vi "SubVI_ShowIncorrectImg_002.vi"(1 "output cluster":T1, 2 "selected path":path[](array[path]), 3 "Correct?":bool[](array[boolean])) -> (0 "This VI":refnum<vi>)   [LabVIEW 2018]
uses:
  <vilib>/picture/picture.llb/Draw 1-Bit Pixmap.vi
panel:
  in  "Close This Window":bool
  out "File name":string[](array[string])
  out "Result given":string[](array[string])
  out "Uncorrectly classified pics":picture[](array[picture])
  in  "Just an empty square. Look away!":picture
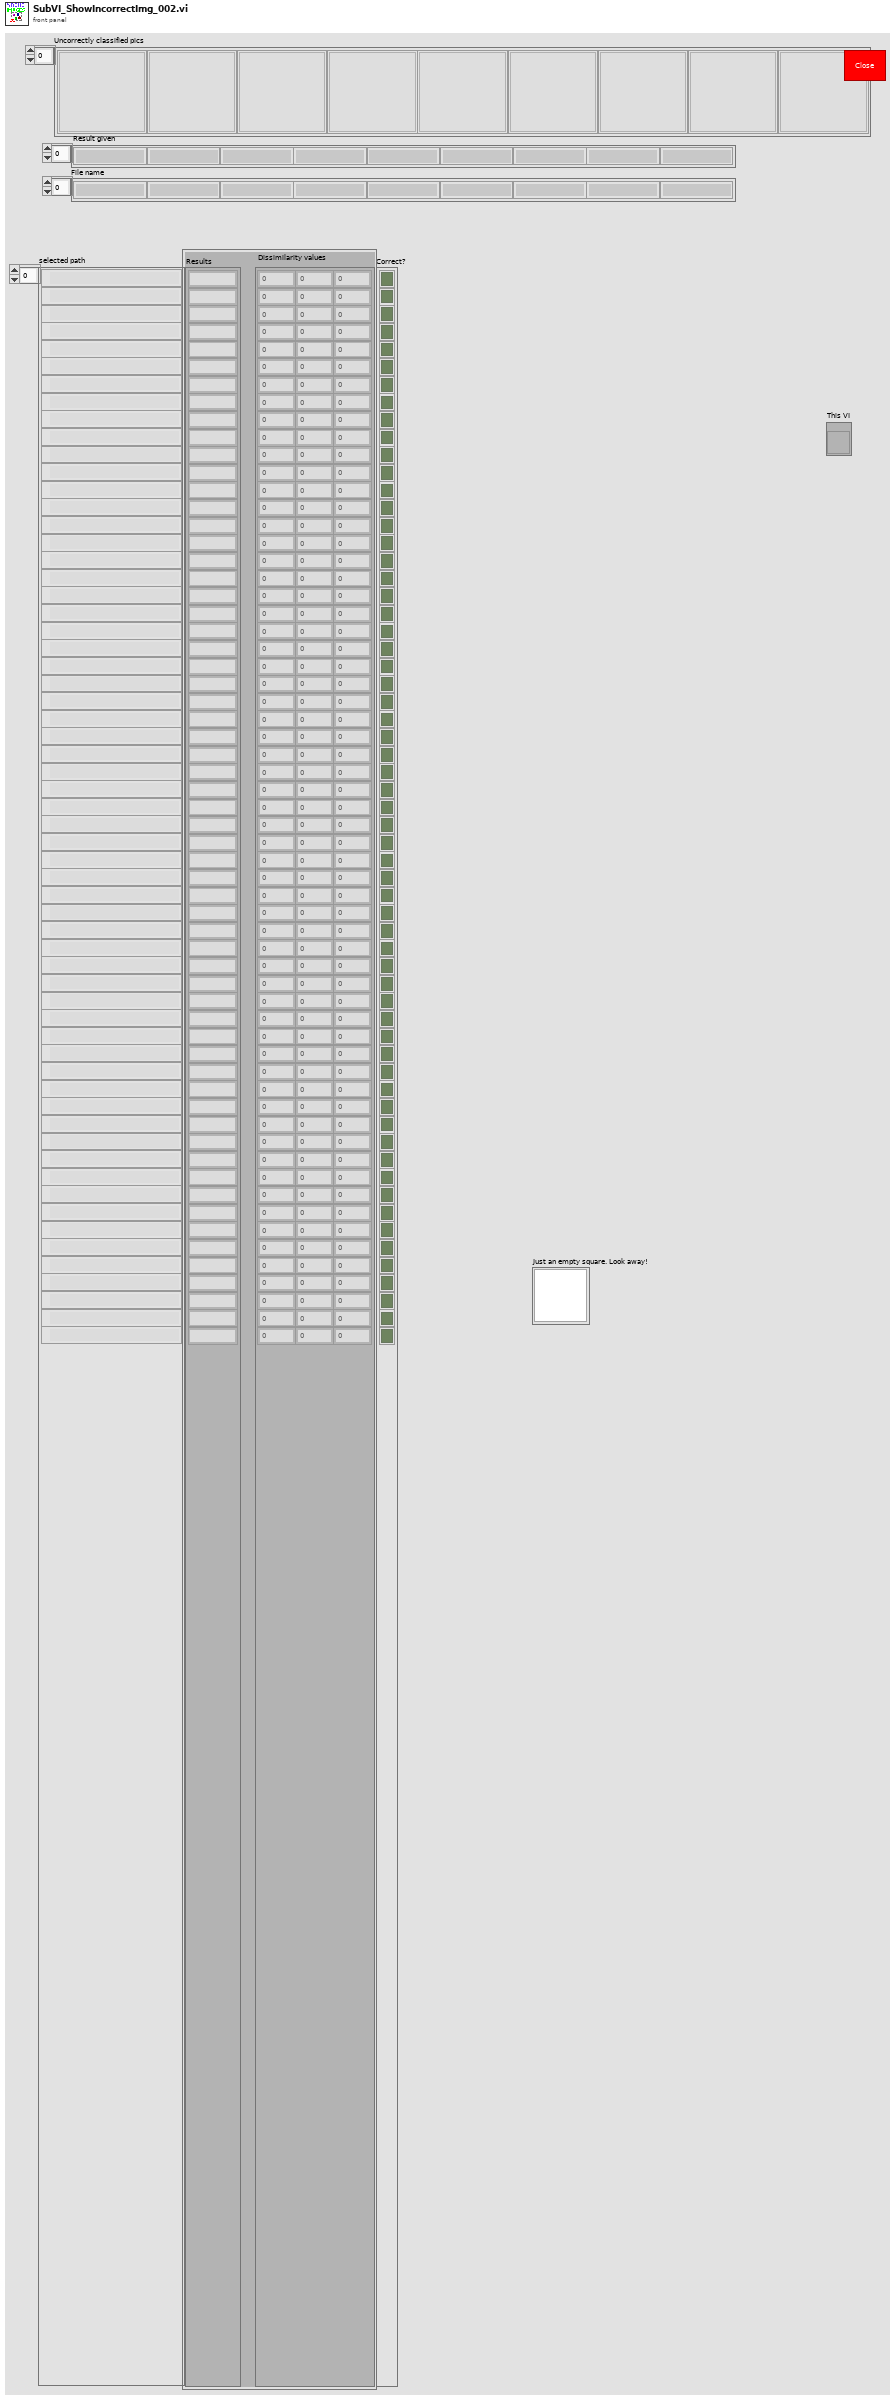
[diagram p1: front panel]
types:
  T1 = cluster{"Results":string[], "Dissimilarity values":dbl[][]}
  T2 = typedef "imagedata.ctl" = cluster{"image type":i32, "image depth":i32, "image":u8[], "mask":u8[], "colors":u32[], "Rectangle":cluster{"left":i16, "top":i16, "right":i16, "bottom":i16}}
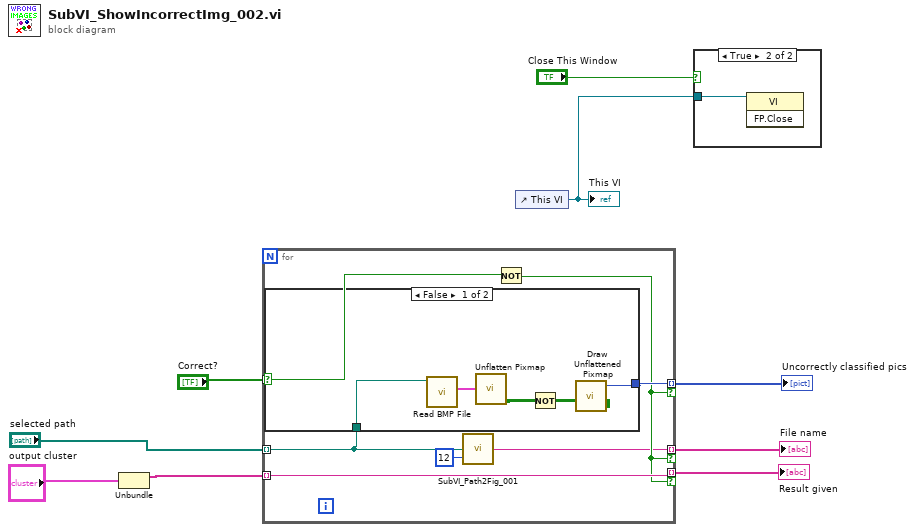
[diagram p0: block diagram]
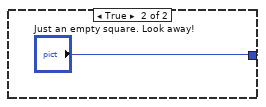
[diagram p3: hidden frame]
diagram:
  n1 = Unbundle("output cluster") -> ("Results"=w4:string[])  [unwired: 1 out]
  n2 = for {
    tunnel: "Correct?" -> [w15] mode=indexing
    tunnel: "selected path" -> [w10] mode=indexing
    tunnel: w4 -> [w14] mode=indexing
    tunnel: [w16] -> w9 mode=indexing if=w13
    tunnel: [w14] -> w8 mode=indexing if=w13
    tunnel: [w12] -> w7 mode=indexing if=w13
    n3 = case shown="False" w15 {
      tunnel: [w19 "Just an empty square. Look away!"] -> w16
      tunnel: w10 -> [w17 _]
      frame False {
        n4 = call <vilib>:"Read BMP File.vi"("path to BMP file"=w17) -> ("image data"=w18:T2)  [unwired: 8 in, 2 out]
        n5 = call <vilib>:"Unflatten Pixmap.vi"("image data"=w18) -> ("1-bit pixmap"=w21:bool[][])  [unwired: 4 in, 6 out]
        n6 = Not(x=w21) -> (.not. x?=w20:bool[][])
        n7 = call-poly <vilib>:"Draw Unflattened Pixmap.vi"("data"=w20) -> ("new picture"=w19:picture)  [unwired: 8 in]
      }
      frame True {
      }
    }
    n8 = call "SubVI_Path2Fig_001.vi"("length (rest)"=12, "Path"=w10) -> ("FIG"=w12:string)
    n9 = Not(x=w15) -> (.not. x?=w13:bool)
  }
  "Uncorrectly classified pics" <- w9
  "Result given" <- w8
  "File name" <- w7
  n10 = control-ref of="This VI"() -> (w6:refnum<vi>)
  "This VI" <- w6
  n11 = case shown="True" "Close This Window" {
    tunnel: w6 -> [_ w23]
    frame False {
    }
    frame True {
      n12 = invoke class="VI" method="FP.Close"(reference=w23) -> ()  [unwired: 2 in, 3 out]
    }
  }
